vi "Dialog Tester - Error Prompt.vi"() -> ()   [LabVIEW 2019]
doc: "<b>TEST VI</b> meant to check formatting of the error prompt"
uses:
  <vilib>/Utility/error.llb/DialogType.ctl
  <vilib>/Utility/error.llb/Error Cluster From Error Code.vi
  <vilib>/ErrorRing/Error Ring.xnode
  Theme/Theme.lvclass
  Standard/Error-Prompt/Error-Prompt.lvclass
panel:
  out "Choice?":bool
  out "error out":errorcluster
  in  "dark?":bool
  in  "Error In":errorcluster
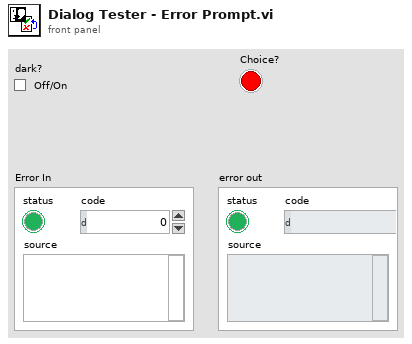
[diagram p1: front panel]
types:
  T1 = typedef "DialogType.ctl" = u16
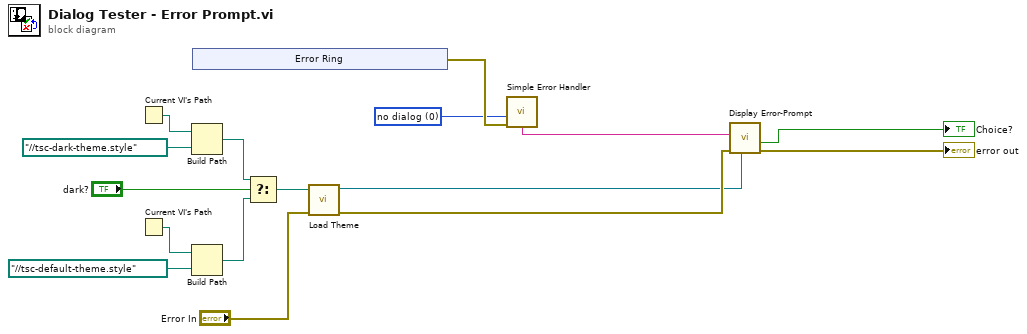
[diagram p0: block diagram]
diagram:
  w2 = T1 0 items=["no dialog", "OK message", "continue or stop message", "OK message + warnings", "continue/stop + warnings"] ("type of dialog (OK msg:1)")
  n1 = Current VI's Path() -> (path=w9:path)
  n2 = Current VI's Path() -> (path=w10:path)
  n3 = Build Path(base path=w9, name or relative path=path "../../tsc-dark-theme.style") -> (appended path=w15:path)
  n4 = Build Path(base path=w10, name or relative path=path "../../tsc-default-theme.style") -> (appended path=w11:path)
  n5 = xnode "Error Ring"() -> ("error out"=w3:errorcluster)
  n6 = Select(t=w15, s="dark?", f=w11) -> (s? t:f=w14:path)
  n7 = call "Load Theme.vi"("error in"="Error In", "File Path"=w14) -> ("error out"=w8:errorcluster, "Theme"=w7:refnum<class "Theme.lvclass">)  [unwired: 8 in]
  n8 = call <vilib>:"Simple Error Handler.vi"("type of dialog (OK msg:1)"=w2, "error in (no error)"=w3) -> ("message"=w1:string)  [unwired: 3 in, 4 out]
  n9 = call "Display Error-Prompt.vi"("Theme"=w7, "error in"=w8, "Error Message"=w1) -> ("error out"=→"error out":errorcluster, "Choice?"=→"Choice?":bool)  [unwired: 7 in]
